vi "Waveform to Reference.vi"(5 "Waveform":cluster{"t0":dbl, "dt":dbl, "y":csg[]}, 12 "error in (no error)":errorcluster) -> (6 "Data":refnum<data-value>, 14 "error out":errorcluster)   [LabVIEW 2016, in "Common.lvlib"]
uses:
  Common.lvlib
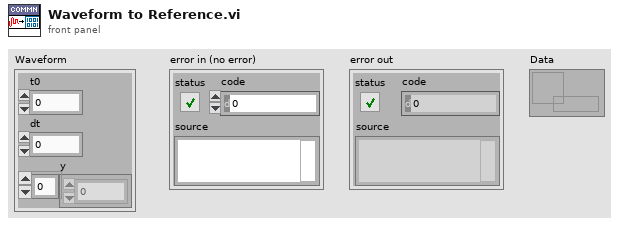
[diagram p1: front panel]
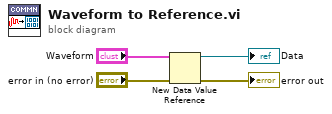
[diagram p0: block diagram]
diagram:
  n1 = New Data Value Reference(data value="Waveform", error in="error in (no error)") -> (data value reference=→"Data":refnum<data-value>, error out=→"error out":errorcluster)
